vi "DOAction.vi"(6 "Slot":T1, 8 "error in":errorcluster, 10 "State":string, 11 "CH":string) -> (0 "error out":errorcluster)   [LabVIEW 2013]
uses:
  SystemCode/SysControl/Slot.ctl
  <vilib>/DAQmx/write.llb/DAQmx Write (Digital Bool 1Line 1Point).vi
  <vilib>/DAQmx/read.llb/DAQmx Read (Digital Bool 1Line 1Point).vi
  SourceCode/GlobalValue.vi
  <vilib>/DAQmx/create/channels.llb/DAQmx Create Channel (DO-Digital Output).vi
  <vilib>/DAQmx/miscellaneous.llb/DAQmx Fill In Error Info.vi
panel:
  out "DO status":bool
  out "State":bool
  out "Line/port":tag="PCI-6229/port0/line0:1"
  in  "Enum":enum16{"Set", "Get", "Initialize"}(ring)
  # "CylinderCtrl"
  # "B+"
  # "ACC"
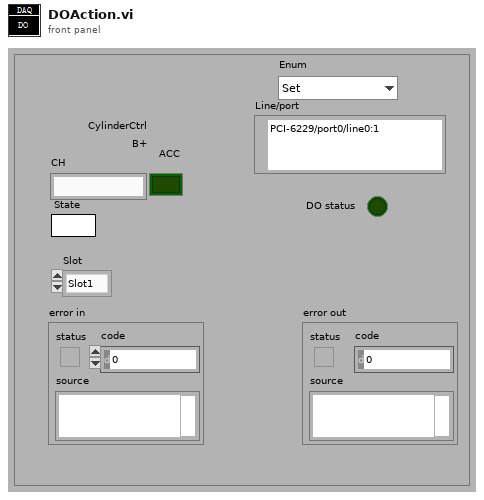
[diagram p1: front panel]
types:
  T1 = typedef "Slot.ctl" = enum16{"Slot1", "Slot2", "Slot3", "Slot4"}
  T2 = typedef "DAQConfig.ctl" = cluster{"DIO":string[][], "AO":string[][], "AI":string[][]}
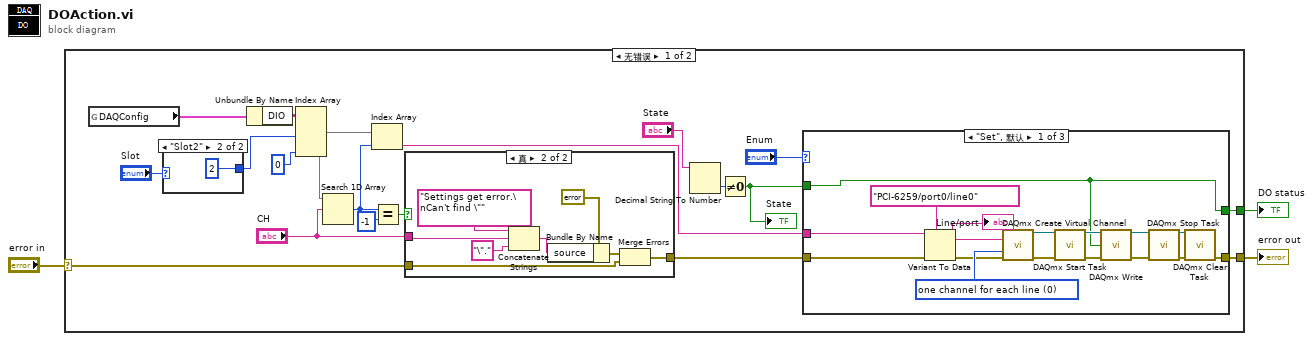
[diagram p0: block diagram]
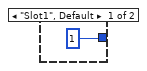
[diagram p2: hidden frame]
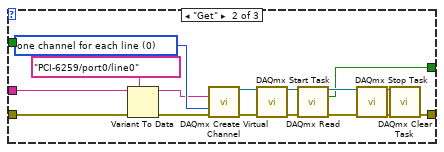
[diagram p4: hidden frame]
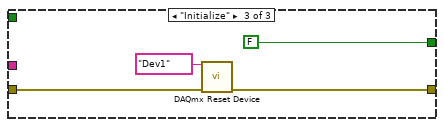
[diagram p5: hidden frame]
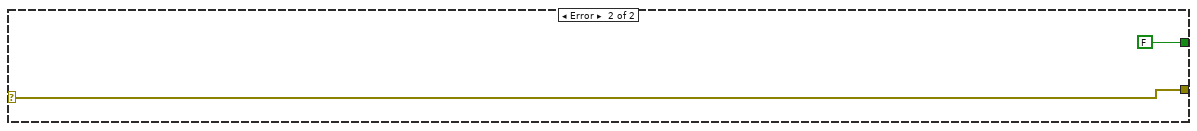
[diagram p6: hidden frame]
diagram:
  n1 = case shown="无错误" "error in" {
    selector: "error in" -> [w7 w72]
    tunnel: [w19 w72] -> w3
    tunnel: [w15 FALSE ("data")] -> w2
    frame No Error {
      n2 = global read "GlobalValue.vi" "DAQConfig"() -> (w4:T2)
      n3 = case shown="\"Slot2\"" "Slot" {
        tunnel: [1 ("索引 (行)") 2 ("索引 (行)")] -> w5
        frame "Slot1", Default {
        }
        frame "Slot2" {
        }
      }
      n4 = Unbundle By Name(w4) -> ("DIO"=w21:string[][])
      n5 = Index Array(array=w21, index (col) #1=w5, index (col) #2=0 ("索引 (列)")) -> (element #1=w9:string[], element #2=w8:string[])  [unwired: 2 in]
      n6 = Search 1D Array(1D array=w8, element="CH") -> (index of element=w18:i32)  [unwired: 1 in]
      n7 = Index Array(array=w9, index=w18) -> (element=w22:string)
      n8 = Equal?(x=w18, y=-1) -> (x = y?=w16:bool)
      n9 = case shown="真" w16 {
        tunnel: "CH" -> [_ w30]
        tunnel: w7 -> [w26 w29]
        tunnel: [w26 w28] -> w14
        frame False {
        }
        frame True {
          n10 = Concatenate Strings("Settings get error.\nCan't find \"" ("message"), w30, "\"." ("string")) -> (w33:string)
          n11 = Bundle By Name(cluster=errorcluster {"status"=TRUE, "code"=5000, "source"=""} ("error in 1 (no error)"), "source"=w33) -> (w32:errorcluster)
          n12 = Merge Errors(w32, w29) -> (w28:errorcluster)
        }
      }
      n13 = Decimal String To Number(string="State") -> (number=w11:i32)  [unwired: 2 in, 1 out]
      n14 = Not Equal To 0?(x=w11) -> (x != 0?=w12:bool)
      "State" <- w12
      n15 = case shown="\"Set\", 默认" "Enum" {
        tunnel: w14 -> [w36 w51 w70]
        tunnel: [w44 w60 w69] -> w19
        tunnel: [w35 w53 FALSE ("data")] -> w15
        tunnel: w22 -> [w37 w52 _]
        tunnel: w12 -> [w35 _ _]
        frame "Set", Default {
          w39 = 0 items=["one channel for each line", "one channel for all lines"] ("line grouping")
          n16 = Variant To Data(error in=w36, type=tag "PCI-6259/port0/line0" ("lines"), Variant=w37) -> (data=w42:tag, error out=w38:errorcluster)
          "Line/port" <- w42
          n17 = call-poly <vilib>:"DAQmx Create Virtual Channel.vi"("lines"=w42, "line grouping"=w39, "error in"=w38) -> ("task out"=w50:refnum<k21>, "error out"=w49:errorcluster)  [unwired: 11 in]
          n18 = call <vilib>:"DAQmx Start Task.vi"("task/channels in"=w50, "error in"=w49) -> ("task out"=w48:refnum<k21>, "error out"=w47:errorcluster)  [unwired: 12 in]
          n19 = call-poly <vilib>:"DAQmx Write.vi"("task/channels in"=w48, "data"=w35, "error in"=w47) -> ("task out"=w41:refnum<k21>, "error out"=w40:errorcluster)  [unwired: 10 in, 1 out]
          n20 = call <vilib>:"DAQmx Stop Task.vi"("task/channels in"=w41, "error in"=w40) -> ("task out"=w46:refnum<k21>, "error out"=w45:errorcluster)  [unwired: 12 in]
          n21 = call <vilib>:"DAQmx Clear Task.vi"("task in"=w46, "error in"=w45) -> ("error out"=w44:errorcluster)  [unwired: 13 in]
        }
        frame "Get" {
          w59 = 0 items=["one channel for each line", "one channel for all lines"] ("line grouping")
          n22 = Variant To Data(error in=w51, type=tag "PCI-6259/port0/line0" ("lines"), Variant=w52) -> (data=w57:tag, error out=w56:errorcluster)
          n23 = call-poly <vilib>:"DAQmx Create Virtual Channel.vi"("lines"=w57, "line grouping"=w59, "error in"=w56) -> ("task out"=w66:refnum<k21>, "error out"=w65:errorcluster)  [unwired: 11 in]
          n24 = call <vilib>:"DAQmx Start Task.vi"("task/channels in"=w66, "error in"=w65) -> ("task out"=w64:refnum<k21>, "error out"=w63:errorcluster)  [unwired: 12 in]
          n25 = call-poly <vilib>:"DAQmx Read.vi"("task/channels in"=w64, "error in"=w63) -> ("task out"=w55:refnum<k21>, "data"=w53:bool, "error out"=w54:errorcluster)  [unwired: 11 in]
          n26 = call <vilib>:"DAQmx Stop Task.vi"("task/channels in"=w55, "error in"=w54) -> ("task out"=w62:refnum<k21>, "error out"=w61:errorcluster)  [unwired: 12 in]
          n27 = call <vilib>:"DAQmx Clear Task.vi"("task in"=w62, "error in"=w61) -> ("error out"=w60:errorcluster)  [unwired: 13 in]
        }
        frame "Initialize" {
          n28 = call <vilib>:"DAQmx Reset Device.vi"("device in"=tag "Dev1", "error in"=w70) -> ("error out"=w69:errorcluster)  [unwired: 13 in]
        }
      }
    }
    frame Error {
    }
  }
  "error out" <- w3
  "DO status" <- w2
